vi "MonoSpec50 Control.vi"(4 "error in (no error)":errorcluster) -> (0 "error out":errorcluster)   [LabVIEW 2012]
doc: "Ce VI permet à l'utilisateur de contrôler la position, en nm, du monochromateur MonoSpec 50.\nIl y est aussi possible de procéder à la saisie d'une nouvelle position actuelle."
uses:
  <vilib>/Utility/error.llb/DialogType.ctl
panel:
  out "Moving":bool caption="Déplacement\nen cours"
  in  "Quitter":bool
  in  "NewPos":bool caption="Entrer une nouvelle\nposition actuelle"
  out "PosAct":dbl caption="Position\nActuelle (nm)"
  in  "PosDem":dbl caption="Position\nDemandée (nm)"
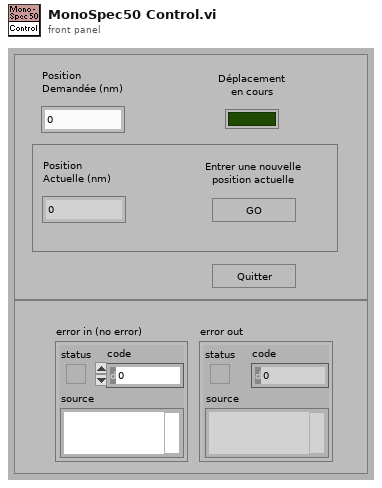
[diagram p1: front panel]
types:
  T1 = typedef "DialogType.ctl" = u16
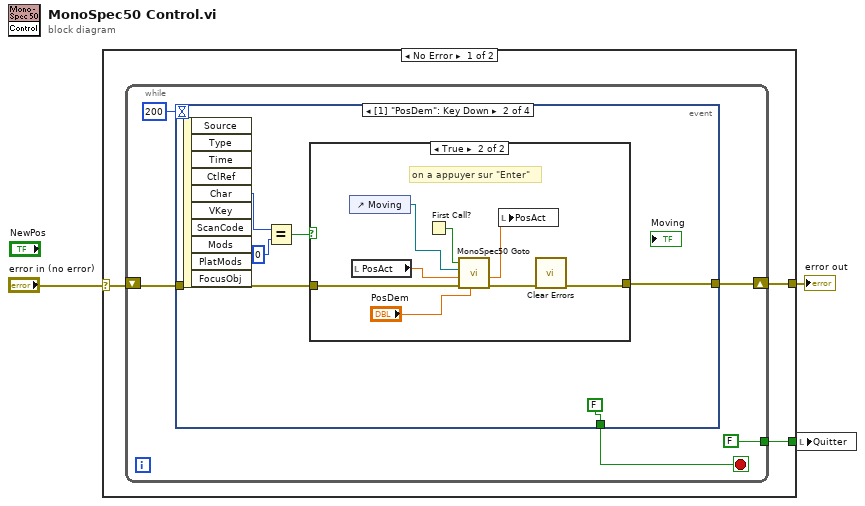
[diagram p0: block diagram]
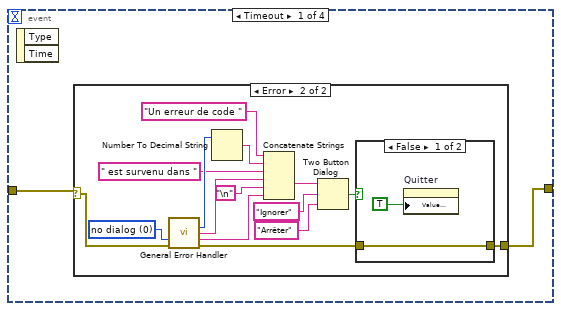
[diagram p2: hidden frame]
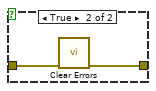
[diagram p4: hidden frame]
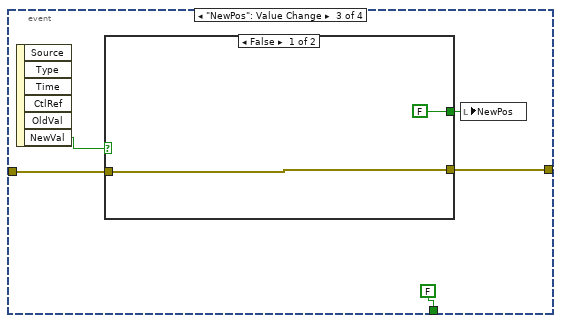
[diagram p6: hidden frame]
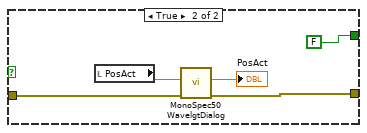
[diagram p7: hidden frame]
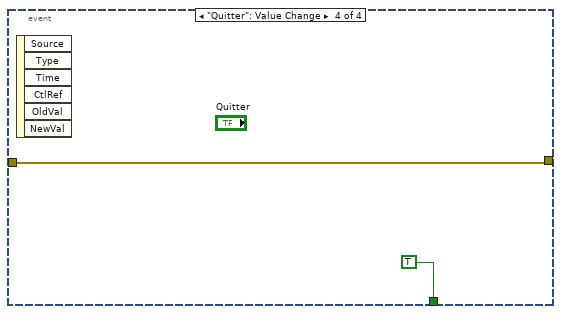
[diagram p8: hidden frame]
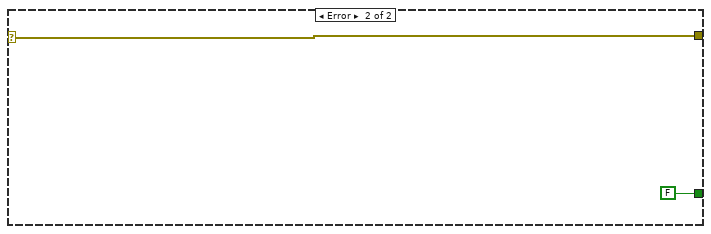
[diagram p9: hidden frame]
diagram:
  n1 = case shown="No Error" "error in (no error)" {
    selector: "error in (no error)" -> [w5 w64]
    tunnel: [w6 w64] -> w2
    tunnel: [w4 FALSE ("Quitter")] -> w1
    frame No Error {
      n2 = while {
        shift-right: [w11] -> w6
        shift-left: w5 -> [w9]
        tunnel: [FALSE ("Quitter")] -> w4
        stop <- w8 stop-if-true
        n3 = event shown="[1] \"PosDem\": Key Down" {
          selector: _ -> [_ _ _ _]
          dyn-events: _ -> [_ _ _ _]
          timeout: 200 -> [_ _ _ _]
          tunnel: [w12 w36 w51 w61] -> w11
          tunnel: w9 -> [w13 w35 w52 w61]
          tunnel: [_ FALSE FALSE TRUE] -> w8
          event Timeout {
            n4 = event-data() -> ()  [unwired: 1 in, 2 out]
            n5 = case shown="Error" w13 {
              selector: w13 -> [w14 w15]
              tunnel: [w14 w16] -> w12
              frame No Error {
              }
              frame Error {
                w26 = T1 0 items=["no dialog", "OK message", "continue or stop message", "OK message + warnings", "continue/stop + warnings"] ("type of dialog (OK msg:1)")
                n6 = call <vilib>:"General Error Handler.vi"("type of dialog (OK msg:1)"=w26, "error in (no error)"=w15) -> ("code out"=w22:i32, "source out"=w21:string, "message"=w19:string, "error out"=w17:errorcluster)  [unwired: 9 in, 1 out]
                n7 = Number To Decimal String(number=w22) -> (decimal integer string=w23:string)  [unwired: 1 in]
                n8 = Concatenate Strings("Un erreur de code " ("string"), w23, " est survenu dans " ("string"), w21, "\n", w19) -> (w18:string)
                n9 = Two Button Dialog(message=w18, 1:"Arrêter" ("F button name (\"Cancel\")"), 2:"Ignorer" ("T button name (\"OK\")")) -> (T button?=w29:bool)
                n10 = case shown="False" w29 {
                  tunnel: w17 -> [w31 w32]
                  tunnel: [w31 w33] -> w16
                  frame False {
                    n11 = property on="Quitter" class="Bool (strict)"("Value (Signaling)"=TRUE) -> ()  [unwired: 2 in, 2 out]
                  }
                  frame True {
                    n12 = call <vilib>:"Clear Errors.vi"("error in (no error)"=w32) -> ("error out"=w33:errorcluster)  [unwired: 6 in]
                  }
                }
              }
            }
          }
          event "PosDem": Key Down {
            n13 = event-data() -> ("Char"=w37:i16)  [unwired: 1 in, 9 out]
            n14 = Equal?(x=w37, y=i16 0) -> (x = y?=w39:bool)
            n15 = case shown="True" w39 {
              tunnel: [w40 w41] -> w36
              tunnel: w35 -> [w40 w48]
              frame False {
              }
              frame True {
                # "on a appuyer sur \"Enter\""
                n16 = control-ref of="Moving"() -> (w44:refnum<vi>)
                n17 = local read "PosAct"() -> (w47:dbl)
                n18 = First Call?() -> (First Call?: T/F=w43:bool)
                n19 = call <userlib>:"MonoSpec50 Goto.vi"("PosDem"="PosDem", "error in (no error)"=w48, "PosAct"=w47, "Moving Ref"=w44, "Ask Act Pos"=w43) -> ("error out"=w42:errorcluster, "PosAct Out"=w46:dbl)  [unwired: 2 in]
                n20 = local write "PosAct"(w46) -> ()
                n21 = call <vilib>:"Clear Errors.vi"("error in (no error)"=w42) -> ("error out"=w41:errorcluster)  [unwired: 6 in]
              }
            }
          }
          event "NewPos": Value Change {
            n22 = event-data() -> ("NewVal"=w53:bool)  [unwired: 1 in, 5 out]
            n23 = case shown="False" w53 {
              tunnel: w52 -> [w55 w60]
              tunnel: [w55 w59] -> w51
              tunnel: [FALSE FALSE] -> w49
              frame False {
              }
              frame True {
                n24 = local read "PosAct"() -> (w57:dbl)
                n25 = call <userlib>:"MonoSpec50 WavelgtDialog.vi"("error in (no error)"=w60, "PosAct"=w57) -> ("error out"=w59:errorcluster, "PosAct Out"=→"PosAct":dbl)  [unwired: 4 in]
              }
            }
            n26 = local write "NewPos"(w49) -> ()
          }
          event "Quitter": Value Change {
            n27 = event-data() -> ()  [unwired: 1 in, 6 out]
          }
        }
      }
    }
    frame Error {
    }
  }
  "error out" <- w2
  n28 = local write "Quitter"(w1) -> ()
